vi "Teleop.vi"(10 "Match Info":T1={"Autonomous Elapsed Seconds"=0.0, "TeleOp Elapsed Seconds"=0.0, "Disabled Elapsed Seconds"=0.0, "Visited Autonomous"=FALSE, "Visited TeleOp"=FALSE, "Visited Disabled"=FALSE, "Autonomous Settings"={"Autonomous Style"=enum."Independent", "VI Refnum"=refnum}}, 11 "Call Context":T2) -> ()   [LabVIEW 2019]
doc: "This VI is called for each enabled TeleOp packet received from the DS. It is typically used to read from joysticks and other inputs and update I/O or setpoints for timed control loops. It should complete and return within 20 milliseconds or risk missing DS packets."
uses:
  <vilib>/Rock Robotics/WPI/DriverStation/WPI_DriverStationDerivedRobotMode.ctl
  <vilib>/Rock Robotics/WPI/DriverStation/WPI_DriverStationMatch Info.ctl
  Drive/Implementation/Drive Operations.ctl
  <vilib>/Rock Robotics/WPI/Utilities/WPI_GetSetVariantRefNum.vi
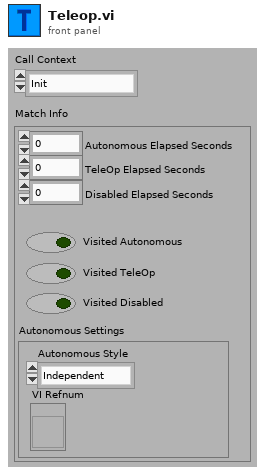
[diagram p1: front panel]
types:
  T1 = typedef "WPI_DriverStationMatch Info.ctl" = cluster{"Autonomous Elapsed Seconds":dbl, "TeleOp Elapsed Seconds":dbl, "Disabled Elapsed Seconds":dbl, "Visited Autonomous":bool, "Visited TeleOp":bool, "Visited Disabled":bool, "Autonomous Settings":cluster{"Autonomous Style":enum16{"Iterative", "Independent"}, "VI Refnum":refnum<vi>}}
  T2 = typedef "WPI_DriverStationDerivedRobotMode.ctl" = enum16{"Init", "Execute", "Stop"}
  T3 = typedef "Drive Operations.ctl" = enum16{"Reserve", "Read Current", "Immediate", "Pod Racer", "Ball AA", "Play Back From Log"}
  T4 = typedef "WPI_JoystickDevRef.ctl" = cluster{"Device":T5}
  T5 = typedef "WPI_JoystickDeviceEnum.ctl" = enum16{"USB 0", "USB 1", "USB 2", "USB 3", "USB 4", "USB 5"}
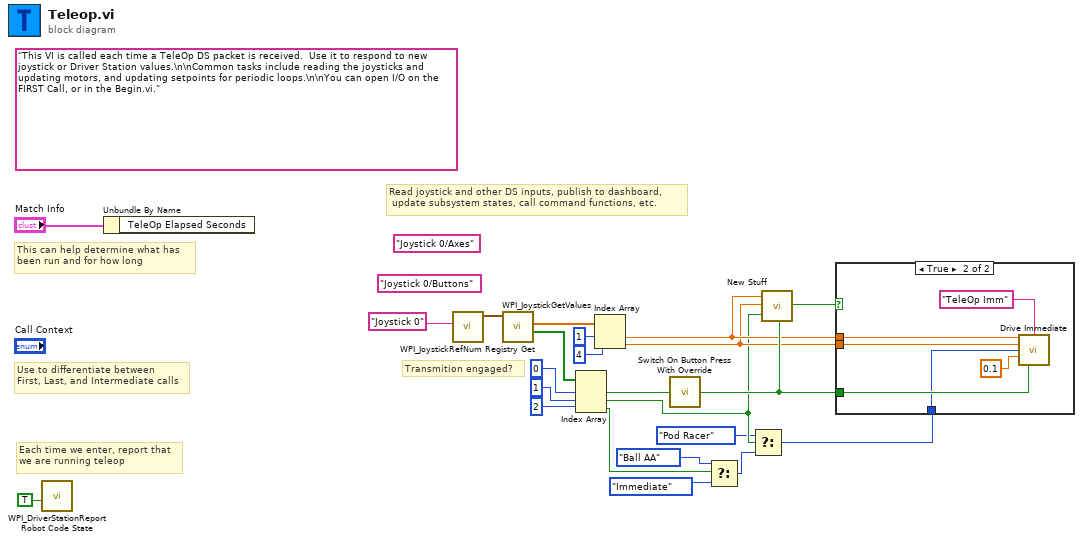
[diagram p0: block diagram]
diagram:
  (unwired) "Joystick 0/Axes" ("Name")
  (unwired) "Joystick 0/Buttons" ("Name")
  (unwired) "This VI is called each time a TeleOp DS packet is received.  Use it to respond to new joystick or Driver Station values.\n\nCommon tasks include reading the joysticks and updating motors, and updating setpoints for periodic loops.\n\nYou can open I/O on the FIRST Call, or in the Begin.vi."
  # "Transmition engaged?"
  # "Read joystick and other DS inputs, publish to dashboard,\n update subsystem states, call command functions, etc."
  # "Each time we enter, report that\nwe are running teleop"
  # "Use to differentiate between\nFirst, Last, and Intermediate calls"
  # "This can help determine what has\nbeen run and for how long"
  n1 = call <vilib>:"WPI_DriverStationReport Robot Code State.vi"("TeleOp"=TRUE ("Autonomous")) -> ()  [unwired: 10 in, 1 out]
  n2 = Unbundle By Name("Match Info") -> ()  [unwired: 1 out]
  n3 = call <vilib>:"WPI_JoystickRefNum Registry Get.vi"("refnum name"="Joystick 0") -> ("JoystickDevRef"=w20:T4)  [unwired: 1 in, 9 out]
  n4 = call <vilib>:"WPI_JoystickGetValues.vi"("JoystickDevRef"=w20) -> ("Buttons"=w17:bool[], "Axes"=w19:dbl[])  [unwired: 6 in, 3 out]
  n5 = Index Array(array=w17, index #1=0 ("index"), index #2=1 ("index"), index #3=2 ("index")) -> (element #1=w15:bool, element #2=w8:bool, element #3=w1:bool)
  n6 = Index Array(array=w19, index #1=1 ("index"), index #2=4 ("index")) -> (element #1=w10:dbl, element #2=w9:dbl)
  n7 = call "Switch On Button Press With Override.vi"("Button"=w15) -> ("Output"=w14:bool)  [unwired: 2 in]
  n8 = Select(t=Drive_Operations."Ball AA" ("Operation"), s=w1, f=Drive_Operations."Immediate" ("Operation")) -> (s? t:f=w6:T3)
  n9 = Select(t=Drive_Operations."Pod Racer" ("Operation"), s=w8, f=w6) -> (s? t:f=w3:T3)
  n10 = call "New Stuff.vi"("Variant 2"=w10, "Variant 3"=w9, "Variant 6"=w8, "Variant 9"=w14) -> ("x != y?"=w18:bool)  [unwired: 23 in]
  n11 = case shown="True" w18 {
    tunnel: w10 -> [_ w28]
    tunnel: w9 -> [_ w27]
    tunnel: w14 -> [_ w26]
    tunnel: w3 -> [_ w24]
    frame False {
    }
    frame True {
      n12 = call "Drive Immediate.vi"("Left Setpoint"=w28, "Description"="TeleOp Imm", "Right Setpoint"=w27, "Operation"=w24, "Deadband Value"=0.1, "Transmition Engaged?"=w26) -> ()  [unwired: 9 in, 1 out]
    }
  }
